vi "PAM Save Spectra.vi"(9 "Time":timestamp, 10 "PSD":dbl[](array[numeric]), 11 "icListen":string="icListen 1") -> ()   [LabVIEW 2020]
panel:
  out "Error Out":errorcluster
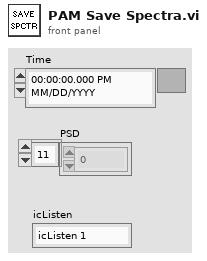
[diagram p1: front panel]
types:
  T1 = enum16{"open", "replace", "create", "open or create", "replace or create", "replace or create with confirmation"}
  T2 = cluster{"Time Window":dbl, "Base Folder Path":path, "Collect Training Frames?":bool}
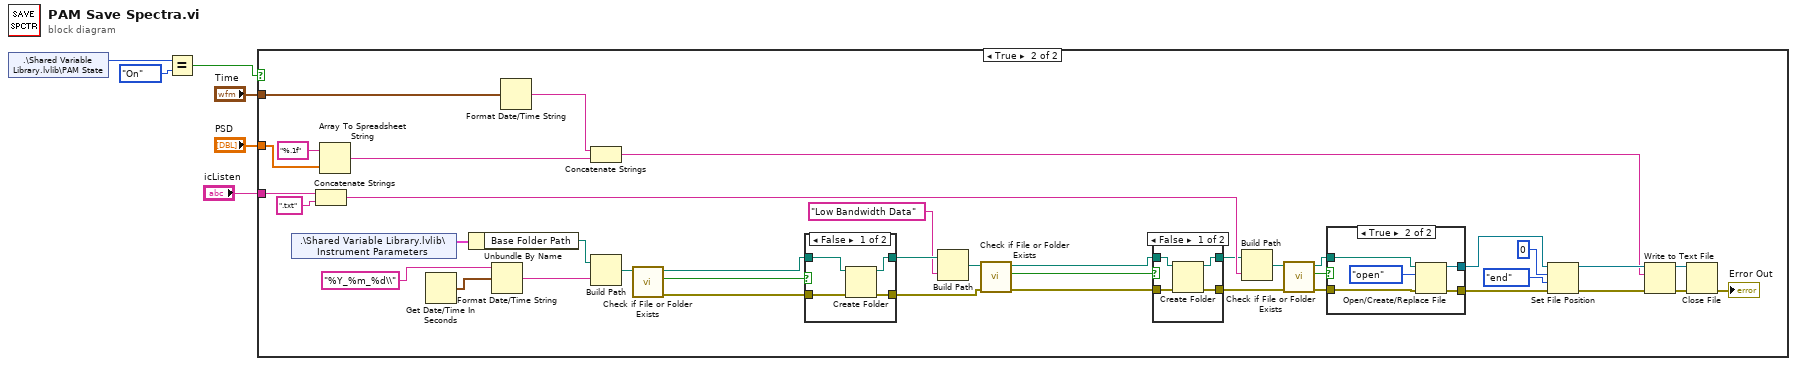
[diagram p0: block diagram]
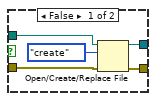
[diagram p3: hidden frame]
diagram:
  n1 = shared-variable ".\\Shared Variable Library.lvlib\\PAM State"() -> (w6:enum16{"Off", "Initialize", "On", "Standby"})  [unwired: 1 in, 1 out]
  n2 = Equal?(x=w6, y=enum16{"Off", "Initialize", "On", "Standby"}."On" ("PAM State")) -> (x = y?=w5:bool)
  n3 = case shown="True" w5 {
    tunnel: "icListen" -> [_ w36]
    tunnel: "Time" -> [_ w35]
    tunnel: "PSD" -> [_ w24]
    frame False {
    }
    frame True {
      n4 = shared-variable ".\\Shared Variable Library.lvlib\\Instrument Parameters"() -> (w40:T2)  [unwired: 1 in, 1 out]
      n5 = Concatenate Strings(w36, ".txt" ("string")) -> (w37:string)
      n6 = Array To Spreadsheet String(array=w24, 3:"%.1f") -> (spreadsheet string=w23:string)  [unwired: 1 in]
      n7 = Get Date/Time In Seconds() -> (seconds since 1Jan1904=w45:timestamp)
      n8 = Unbundle By Name(w40) -> ("Base Folder Path"=w39:path)
      n9 = Format Date/Time String(time format string (%c)="%Y_%m_%d\\", seconds (now)=w45) -> (date/time string=w46:string)  [unwired: 1 in]
      n10 = Format Date/Time String(seconds (now)=w35) -> (date/time string=w22:string)  [unwired: 2 in]
      n11 = Concatenate Strings(w22, w23) -> (w7:string)
      n12 = Build Path(base path=w39, name or relative path=w46) -> (appended path=w43:path)
      n13 = call <vilib>:"Check if File or Folder Exists.vi"("path"=w43) -> ("error out"=w38:errorcluster, "file or folder exists?"=w42:bool, "dup path"=w41:path)  [unwired: 8 in]
      n14 = case shown="False" w42 {
        tunnel: w41 -> [w66 w68]
        tunnel: [w65 w68] -> w29
        tunnel: w38 -> [w64 w67]
        tunnel: [w63 w67] -> w27
        frame False {
          n15 = Create Folder(path (use dialog)=w66, error in=w64) -> (created path=w65:path, error out=w63:errorcluster)  [unwired: 1 in, 1 out]
        }
        frame True {
        }
      }
      n16 = Build Path(base path=w29, name or relative path="Low Bandwidth Data") -> (appended path=w31:path)
      n17 = call <vilib>:"Check if File or Folder Exists.vi"("error in (no error)"=w27, "path"=w31) -> ("error out"=w34:errorcluster, "file or folder exists?"=w32:bool, "dup path"=w33:path)  [unwired: 7 in]
      n18 = case shown="False" w32 {
        tunnel: w33 -> [w60 w62]
        tunnel: [w59 w62] -> w30
        tunnel: w34 -> [w58 w61]
        tunnel: [w57 w61] -> w18
        frame False {
          n19 = Create Folder(path (use dialog)=w60, error in=w58) -> (created path=w59:path, error out=w57:errorcluster)  [unwired: 1 in, 1 out]
        }
        frame True {
        }
      }
      n20 = Build Path(base path=w30, name or relative path=w37) -> (appended path=w17:path)
      n21 = call <vilib>:"Check if File or Folder Exists.vi"("error in (no error)"=w18, "path"=w17) -> ("error out"=w21:errorcluster, "file or folder exists?"=w19:bool, "dup path"=w20:path)  [unwired: 7 in]
      n22 = case shown="True" w19 {
        tunnel: w20 -> [w51 w56]
        tunnel: w21 -> [w49 w54]
        tunnel: [w48 w53] -> w9
        tunnel: [w47 w52] -> w8
        frame False {
          n23 = Open/Create/Replace File(file path (use dialog)=w51, error in=w49, operation (0:open)=T1."create") -> (refnum out=w48:refnum<file>, error out=w47:errorcluster)  [unwired: 3 in, 1 out]
        }
        frame True {
          n24 = Open/Create/Replace File(file path (use dialog)=w56, error in=w54, operation (0:open)=T1."open") -> (refnum out=w53:refnum<file>, error out=w52:errorcluster)  [unwired: 3 in, 1 out]
        }
      }
      n25 = Set File Position(offset (in bytes) (0)=i64 0, refnum=w9, from (0:start)=enum16{"start", "end", "current"}."end", error in=w8) -> (refnum out=w12:refnum<file>, error out=w16:errorcluster)
      n26 = Write to Text File(file (use dialog)=w12, text=w7, error in=w16) -> (refnum out=w14:refnum<file>, error out=w13:errorcluster)  [unwired: 1 in, 1 out]
      n27 = Close File(refnum=w14, error in=w13) -> (error out=→"Error Out":errorcluster)  [unwired: 1 out]
    }
  }
